vi "curve_max.vi"(10 "Ymax":sgl, 11 "Curve in":cluster{"X":dbl[], "Y":dbl[]}) -> (2 "Xc":sgl)   [LabVIEW 2011]
uses:
  <vilib>/gmath/NI_Gmath.lvlib
panel:
  # "Given a cluster of X and Y value (as for XY graph), interpolate the critical value of X that a specified Y limit occurs.  It is assumed that the limit occurs in the direction of increasing X."
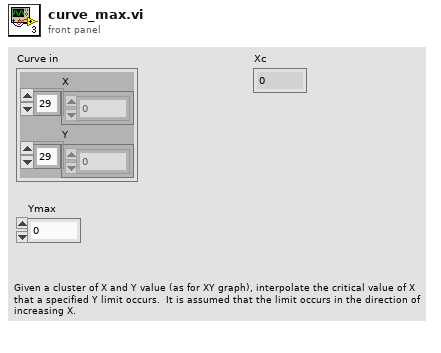
[diagram p1: front panel]
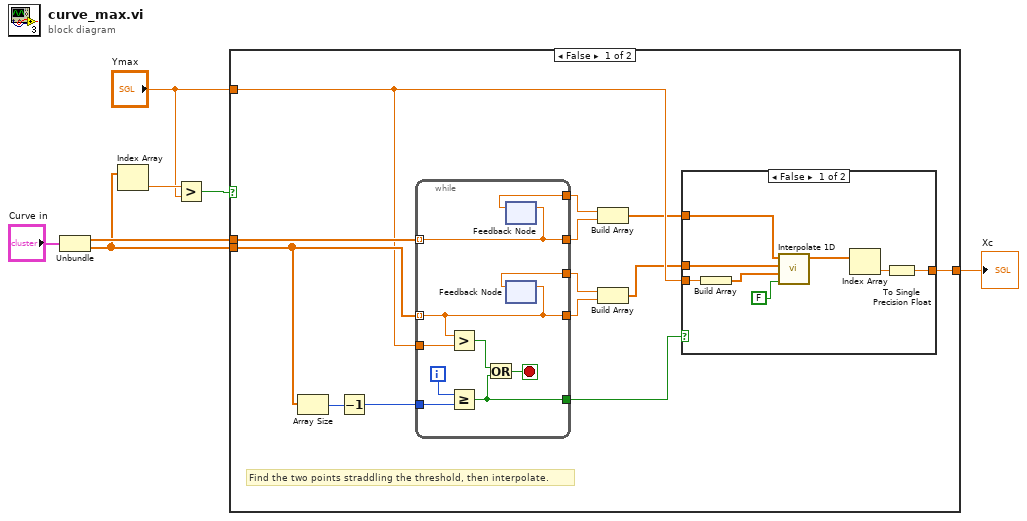
[diagram p0: block diagram]
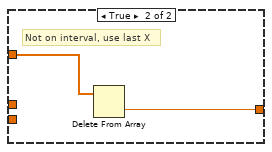
[diagram p2: hidden frame]
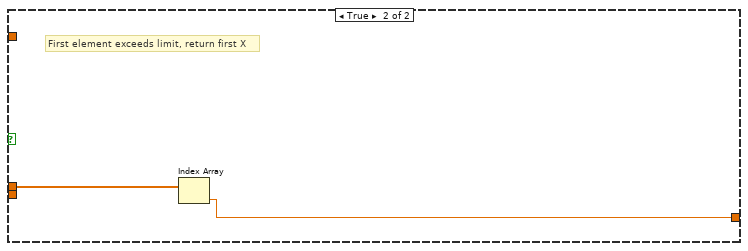
[diagram p3: hidden frame]
diagram:
  n1 = Unbundle("Curve in") -> ("X"=w6:dbl[], "Y"=w4:dbl[])
  n2 = Index Array(array=w4) -> (element=w3:dbl)  [unwired: 1 in]
  n3 = Greater?(x=w3, y="Ymax") -> (0:w1:bool)
  n4 = case shown="False" w1 {
    tunnel: w6 -> [w20 w42]
    tunnel: [w19 w41] -> w5
    tunnel: w4 -> [w15 _]
    tunnel: "Ymax" -> [w14 _]
    frame False {
      # "Find the two points straddling the threshold, then interpolate."
      n5 = Array Size(array=w15) -> (size(s)=w18:i32)
      n6 = Decrement(x=w18) -> (x-1=w17:i32)
      n7 = while {
        tunnel: w20 -> [w34] mode=indexing
        tunnel: w15 -> [w32] mode=indexing
        tunnel: w14 -> [w40]
        tunnel: [w32] -> w10
        tunnel: w17 -> [w37]
        tunnel: [w35] -> w16
        tunnel: [w34] -> w12
        tunnel: [w33] -> w13
        tunnel: [w31] -> w11
        i -> [w36]
        stop <- w38 stop-if-true
        n8 = Greater?(x=w32, y=w40) -> (0:w39:bool)
        n9 = Greater Or Equal?(x=w36, y=w37) -> (x >= y?=w35:bool)
        n10 = Or(x=w39, y=w35) -> (x .or. y?=w38:bool)
        n11 = feedback-in #1(w34) -> ()
        n12 = feedback #1() -> (w33:dbl)  [unwired: 1 in]
        n13 = feedback #2() -> (w31:dbl)  [unwired: 1 in]
        n14 = feedback-in #2(w32) -> ()
      }
      n15 = Build Array(w13, w12) -> (w8:dbl[])
      n16 = Build Array(w11, w10) -> (w9:dbl[])
      n17 = case shown="False" w16 {
        tunnel: w14 -> [w24 _]
        tunnel: [w23 w30] -> w19
        tunnel: w9 -> [w22 _]
        tunnel: w8 -> [w21 w29]
        frame False {
          n18 = Build Array(w24) -> (w25:sgl[])
          n19 = call <vilib>:"Interpolate 1D.vi"("X is monotonic"=FALSE, "xi"=w25, "X"=w22, "Y"=w21) -> ("yi"=w27:dbl[])  [unwired: 5 in, 2 out]
          n20 = Index Array(array=w27) -> (element=w28:dbl)  [unwired: 1 in]
          n21 = To Single Precision Float(number=w28) -> (single precision float=w23:sgl)
        }
        frame True {
          # "Not on interval, use last X"
          n22 = Delete From Array(array=w29) -> (deleted portion=w30:dbl)  [unwired: 2 in, 1 out]
        }
      }
    }
    frame True {
      # "First element exceeds limit, return first X"
      n23 = Index Array(array=w42) -> (element=w41:dbl)  [unwired: 1 in]
    }
  }
  "Xc" <- w5
